vi "Position_Test.vi"() -> ()   [LabVIEW 2015, in "WordManipulationTests.lvlib"]
uses:
  WordManipulationTests.lvlib
  async/WordManipulationLibrary.lvlib
panel:
  out "logical OR":bool
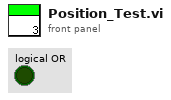
[diagram p1: front panel]
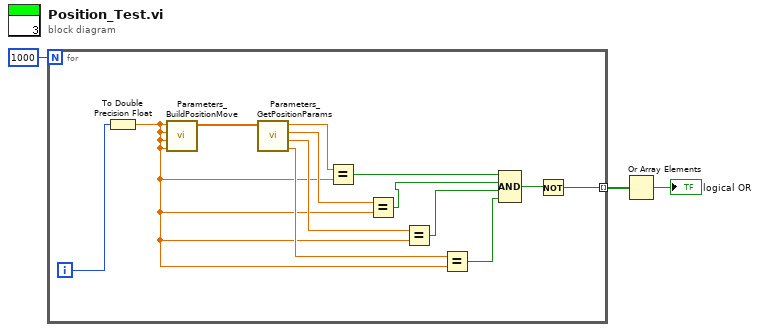
[diagram p0: block diagram]
diagram:
  n1 = for {
    N: 1000 -> [_]
    tunnel: [w4] -> w2 mode=indexing
    i -> [w15]
    n2 = To Double Precision Float(number=w15) -> (double precision float=w10:dbl)
    n3 = call "Parameters_BuildPositionMove.vi"("Acceleration Jerk"=w10, "Acceleration"=w10, "Velocity"=w10, "Target Position"=w10) -> ("Parameters"=w16:dbl[])  [unwired: 7 in]
    n4 = call "Parameters_GetPositionParams.vi"("Parameters"=w16) -> ("Acceleration Jerk"=w11:dbl, "Acceleration"=w12:dbl, "Velocity"=w13:dbl, "Target Position"=w14:dbl)  [unwired: 7 in]
    n5 = Equal?(x=w14, y=w10) -> (x = y?=w9:bool)
    n6 = Equal?(x=w13, y=w10) -> (x = y?=w8:bool)
    n7 = Equal?(x=w12, y=w10) -> (x = y?=w7:bool)
    n8 = Equal?(x=w11, y=w10) -> (x = y?=w6:bool)
    n9 = Compound Arithmetic op=AND(w9, w8, w7, w6) -> (w5:bool)
    n10 = Not(x=w5) -> (.not. x?=w4:bool)
  }
  n11 = Or Array Elements(Boolean array=w2) -> (logical OR=→"logical OR":bool)
